vi "Msg MCLstBox Append.vi"(6 "Username (max 15 characters)":string, 7 "Show Date in LstBox":bool, 8 "error in (no error)":errorcluster, 9 "File Ref":refnum<file>, 10 "Msg":string, 11 "MCListbox Refnum":refnum<vi>) -> (0 "error out":errorcluster)   [LabVIEW 2016, in "Common.lvlib"]
uses:
  <userlib>/Common Components/Common/Common.lvlib
panel:
  # "3 columns if username is not empty\n2 columns otherwise"
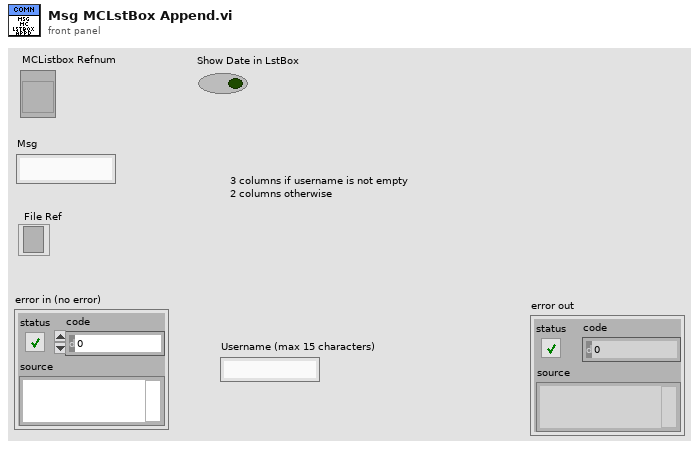
[diagram p1: front panel]
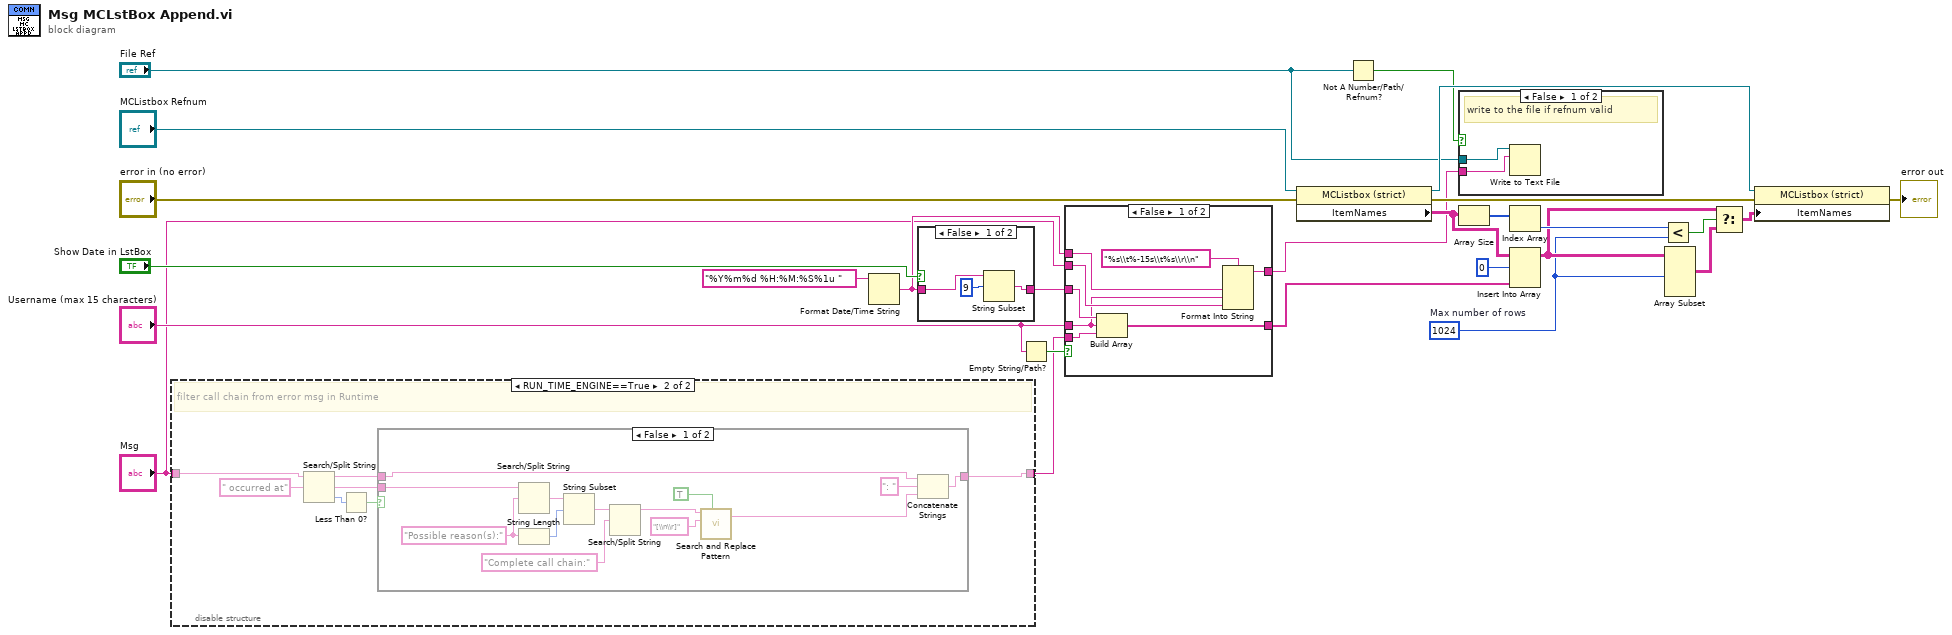
[diagram p0: block diagram]
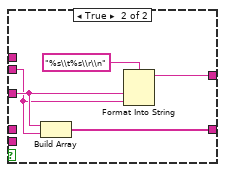
[diagram p4: hidden frame]
diagram:
  w10 = 1024  # Max number of rows
  n1 = disable-structure shown="RUN_TIME_ENGINE==True" {
    disable-tunnel: "Msg" -> [w27 w31]
    disable-tunnel: [w27 w30] -> w1
    frame condition #0 (active) {
    }
    frame condition #1 {
      # "filter call chain from error msg in Runtime"
      n2 = Search/Split String(string=w31, search string/char (-)=" occurred at") -> (substring before match=w32:string, match + rest of string=w33:string, offset of match=w29:i32)  [unwired: 1 in]
      n3 = Less Than 0?(x=w29) -> (x < 0?=w28:bool)
      n4 = case shown="False" w28 {
        tunnel: w33 -> [w47 _]
        tunnel: w32 -> [w41 w48]
        tunnel: [w35 w48] -> w30
        frame False {
          w43 = "Possible reason(s):" ("search string/char (-)")
          n5 = Search/Split String(string=w47, search string/char (-)=w43) -> (match + rest of string=w46:string)  [unwired: 1 in, 2 out]
          n6 = String Length(string=w43) -> (length=w42:i32)
          n7 = String Subset(string=w46, offset (0)=w42) -> (substring=w44:string)  [unwired: 1 in]
          n8 = Search/Split String(string=w44, search string/char (-)="Complete call chain:") -> (substring before match=w39:string)  [unwired: 1 in, 2 out]
          n9 = call <vilib>:"Search and Replace Pattern.vi"("string"=w39, "regular expression (\"\")"="[\\n\\r]" ("regular expression (\"\")"), "replace all? (F)"=TRUE) -> ("result string"=w36:string)  [unwired: 2 in, 1 out]
          n10 = Concatenate Strings(w41, ": " ("string"), w36) -> (w35:string)
        }
        frame True {
        }
      }
    }
  }
  n11 = Format Date/Time String(time format string (%c)="%Y%m%d %H:%M:%S%1u ") -> (date/time string=w6:string)  [unwired: 2 in]
  n12 = case shown="False" "Show Date in LstBox" {
    tunnel: w6 -> [w51 w52]
    tunnel: [w49 w52] -> w8
    frame False {
      n13 = String Subset(string=w51, offset (0)=9) -> (substring=w49:string)  [unwired: 1 in]
    }
    frame True {
    }
  }
  n14 = Empty String/Path?(string/path="Username (max 15 characters)") -> (empty?=w3:bool)
  n15 = case shown="False" w3 {
    tunnel: [w60 w63] -> w16
    tunnel: w8 -> [w59 w62]
    tunnel: w6 -> [w57 _]
    tunnel: "Msg" -> [w56 w61]
    tunnel: [w55 w64] -> w5
    tunnel: "Username (max 15 characters)" -> [w54 _]
    tunnel: w1 -> [w53 _]
    frame False {
      n16 = Build Array(w59, w54, w53) -> (w60:string[])
      n17 = Format Into String(format string="%s\\t%-15s\\t%s\\r\\n", w57, w54, w56) -> (resulting string=w55:string)  [unwired: 2 in, 1 out]
    }
    frame True {
      n18 = Build Array(w62, w61) -> (w63:string[])
      n19 = Format Into String(format string="%s\\t%s\\r\\n", w62, w61) -> (resulting string=w64:string)  [unwired: 2 in, 1 out]
    }
  }
  n20 = property class="MCListbox (strict)"(reference="MCListbox Refnum", error in="error in (no error)") -> (reference out=w25:refnum<vi>, error out=w22:errorcluster, "ItemNames"=w20:string[][])
  n21 = Not A Number/Path/Refnum?(number/path/refnum="File Ref") -> (NaN/Path/Refnum?=w18:bool)
  n22 = case shown="False" w18 {
    tunnel: "File Ref" -> [w67 _]
    tunnel: w5 -> [w66 _]
    frame False {
      # "write to the file if refnum valid"
      n23 = Write to Text File(file (use dialog)=w67, text=w66) -> ()  [unwired: 2 in, 3 out]
    }
    frame True {
    }
  }
  n24 = Array Size(array=w20) -> (size(s)=w19:i32[])
  n25 = Index Array(array=w19) -> (element=w15:i32)  [unwired: 1 in]
  n26 = Insert Into Array(array=w20, index (row)=0 ("index"), new element=w16) -> (w11:string[][])  [unwired: 1 in]
  n27 = Less?(x=w15, y=w10) -> (x < y?=w13:bool)
  n28 = Array Subset(array=w11, length (row)=w10) -> (w9:string[][])  [unwired: 3 in]
  n29 = Select(t=w11, s=w13, f=w9) -> (s? t:f=w12:string[][])
  n30 = property class="MCListbox (strict)"(reference=w25, error in=w22, "ItemNames"=w12) -> (error out=→"error out":errorcluster)  [unwired: 1 out]
